vi "Settings Dialog.vi"(8 "error in (no error)":errorcluster, 11 "Settings in":T1 {"Voltage Limit" scale=0.0..155.0 scale format="%.3g"; "Hardware Configuration"."Baud Rate" items=["<0>"=0, "4800"=4800, "9600"=9600, "19200"=19200, "38400"=38400, "57600"=57600, "115200"=115200]}) -> (0 "error out":errorcluster, 1 "Cancelled?":bool, 2 "UI Refresh Needed?":bool, 3 "Settings out":T1 {"Voltage Limit" scale=0.0..155.0 scale format="%.3g"; "Hardware Configuration"."Baud Rate" items=["<0>"=0, "4800"=4800, "9600"=9600, "19200"=19200, "38400"=38400, "57600"=57600, "115200"=115200]})   [LabVIEW 2022 SP3, in "Settings.lvlib"]
doc: "Dialog for selecting user specified settings."
uses:
  Settings.lvlib
  Settings.ctl
  Acquisition/Hardware Configuration.ctl
  Logging/Logging Configuration.ctl
  <vilib>/Utility/xml.llb/Write to XML File(string).vi
  Acquisition/Acquisition.lvlib
  Logging/Logging.lvlib
panel:
  in  "Reset on Connect":bool
  in  "VISA resource name":refnum<visa-resource-name>
  in  "Baud Rate":u32(ring) items=["<0>"=0, "4800"=4800, "9600"=9600, "19200"=19200, "38400"=38400, "57600"=57600, "115200"=115200]
  in  "Cancel":bool
  in  "OK Button":bool
  # "Non visible portion of dialog (needed for connector pane)."
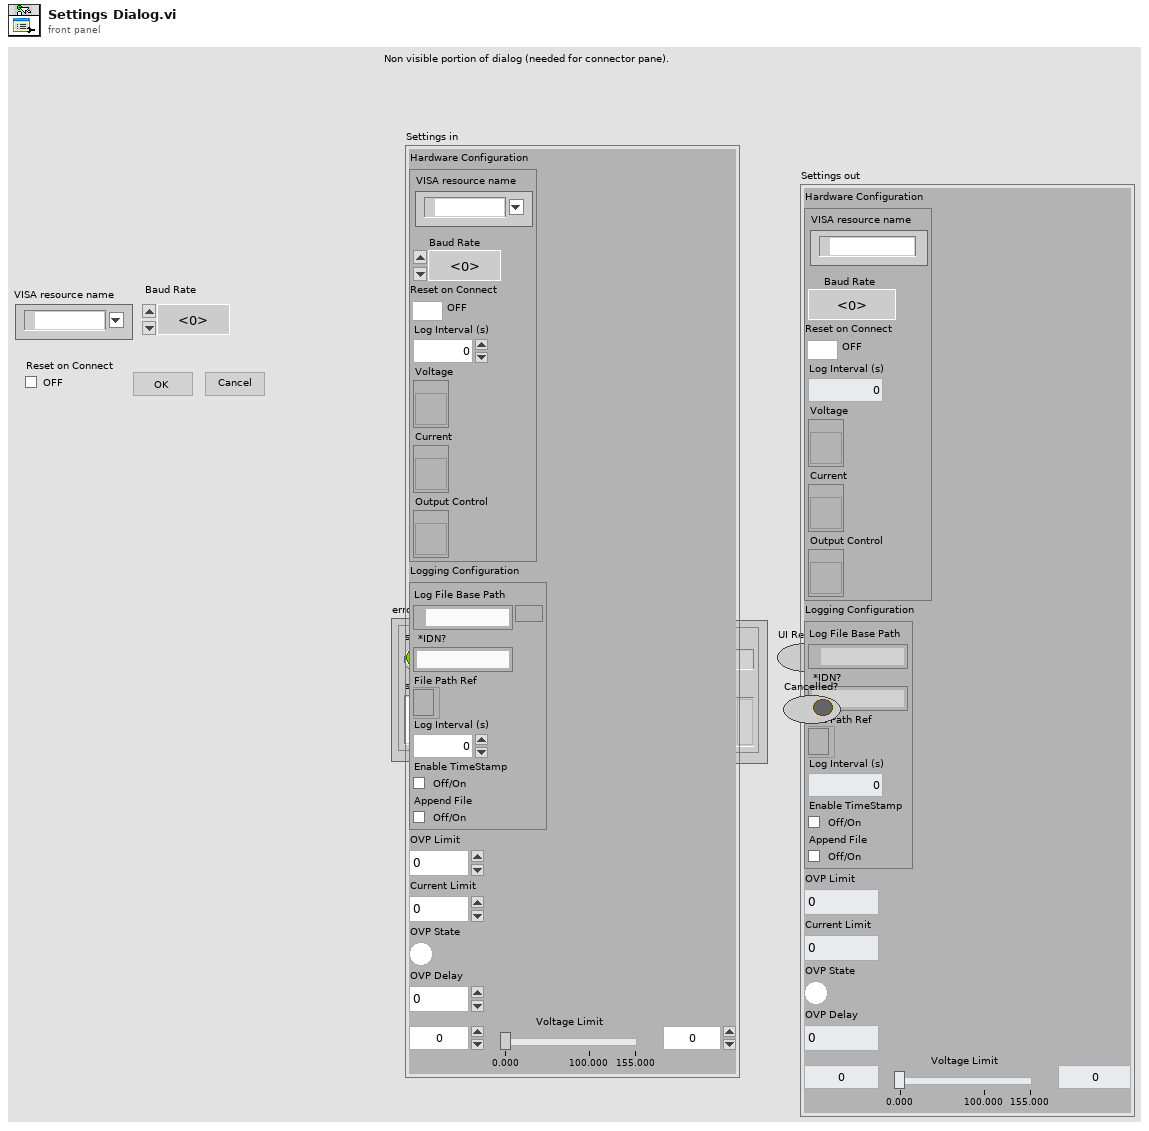
[diagram p1: front panel]
types:
  T1 = typedef "Settings.lvlib/Settings.ctl" = cluster{"Hardware Configuration":T2, "Logging Configuration":T3, "OVP Limit":dbl, "Current Limit":dbl, "OVP State":bool, "OVP Delay":dbl, "Voltage Limit":cluster{"Numeric":dbl, "Numeric":dbl}}
  T2 = typedef "Acquisition.lvlib/Hardware Configuration.ctl" = cluster{"VISA resource name":refnum<visa-resource-name>, "Baud Rate":u32, "Reset on Connect":bool, "Log Interval (s)":dbl, "Voltage":refnum<vi>, "Current":refnum<vi>, "Output Control":refnum<vi>}
  T3 = typedef "Logging.lvlib/Logging Configuration.ctl" = cluster{"Log File Base Path":path, "*IDN?":string, "File Path Ref":refnum<file>, "Log Interval (s)":dbl, "Enable TimeStamp":bool, "Append File":bool}
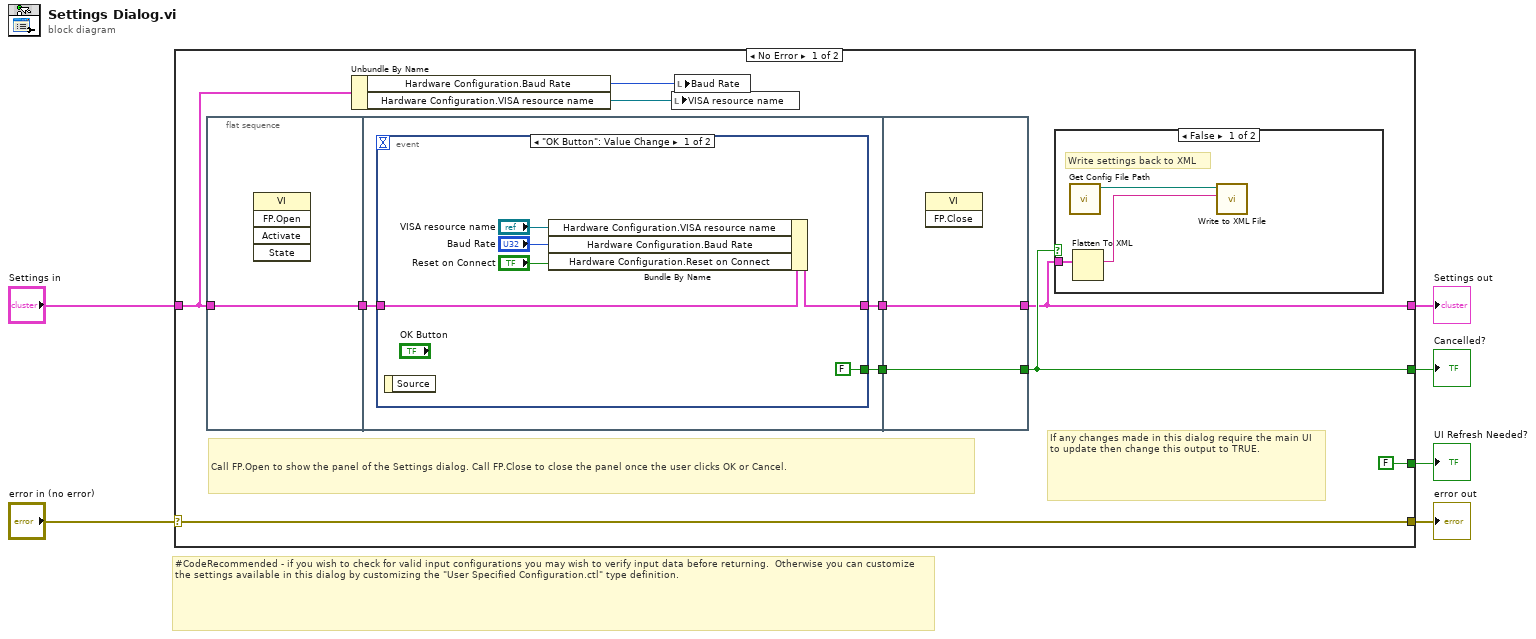
[diagram p0: block diagram]
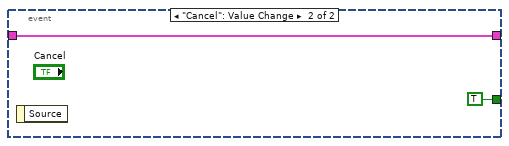
[diagram p2: hidden frame]
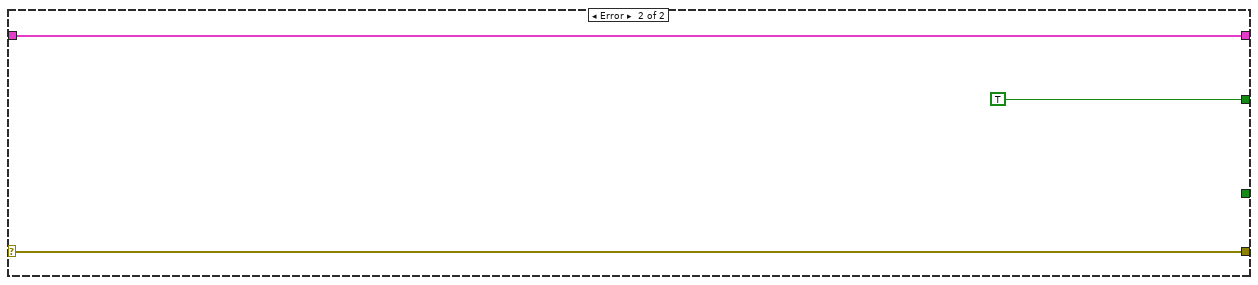
[diagram p4: hidden frame]
diagram:
  # "#CodeRecommended - if you wish to check for valid input configurations you may wish to verify input data before returning.  Otherwise you can customize the settings available in this dialog by customizing the \"User Specified Configuration.ctl\" type definition."
  n1 = case shown="No Error" "error in (no error)" {
    selector: "error in (no error)" -> [w16 w36]
    tunnel: [w16 w36] -> w5
    tunnel: "Settings in" -> [w12 w35]
    tunnel: [w13 w35] -> w3
    tunnel: [FALSE ("UI Refresh Needed?") _] -> w2
    tunnel: [w14 TRUE ("UI Refresh Needed?")] -> w1
    frame No Error {
      # "Call FP.Open to show the panel of the Settings dialog. Call FP.Close to close the panel once the user clicks OK or Cancel."
      # "If any changes made in this dialog require the main UI to update then change this output to TRUE."
      n2 = flat-sequence {
        tunnel: w12 -> [w17]
        tunnel: [w17] -> w11
        tunnel: w11 -> [w18]
        tunnel: [w20] -> w10
        tunnel: [w19] -> w9
        tunnel: [w29] -> w13
        tunnel: [w30] -> w14
        tunnel: w10 -> [w30]
        tunnel: w9 -> [w29]
        frame #0 {
          n3 = invoke class="VI" method="FP.Open"() -> ()  [unwired: 5 in, 5 out]
        }
        frame #1 {
          n4 = event shown="[0] \"OK Button\": Value Change" {
            selector: _ -> [_ _]
            dyn-events: _ -> [_ _]
            timeout: _ -> [_ _]
            tunnel: [w24 w28] -> w19
            tunnel: w18 -> [w25 w28]
            tunnel: [FALSE ("UI Refresh Needed?") TRUE ("UI Refresh Needed?")] -> w20
            event "OK Button": Value Change {
              n5 = event-data() -> ()  [unwired: 1 in, 1 out]
              n6 = Bundle By Name(cluster=w25, "Hardware Configuration.VISA resource name"="VISA resource name", "Hardware Configuration.Baud Rate"="Baud Rate", "Hardware Configuration.Reset on Connect"="Reset on Connect") -> (w24:T1)
            }
            event "Cancel": Value Change {
              n7 = event-data() -> ()  [unwired: 1 in, 1 out]
            }
          }
        }
        frame #2 {
          n8 = invoke class="VI" method="FP.Close"() -> ()  [unwired: 3 in, 3 out]
        }
      }
      n9 = Unbundle By Name(w12) -> ("Hardware Configuration.Baud Rate"=w8:u32, "Hardware Configuration.VISA resource name"=w7:refnum<visa-resource-name>)
      n10 = local write "VISA resource name"(w7) -> ()
      n11 = local write "Baud Rate"(w8) -> ()
      n12 = case shown="False" w14 {
        tunnel: w13 -> [w32 _]
        frame False {
          # "Write settings back to XML"
          n13 = call "Get Config File Path.vi"() -> ("XML File Path"=w33:path)  [unwired: 10 in, 1 out]
          n14 = Flatten To XML(6:w32) -> (2:w31:string)
          n15 = call-poly <vilib>:"Write to XML File.vi"("XML Input"=w31, "XML File Path"=w33) -> ()  [unwired: 7 in, 3 out]
        }
        frame True {
        }
      }
    }
    frame Error {
    }
  }
  "UI Refresh Needed?" <- w2
  "error out" <- w5
  "Settings out" <- w3
  "Cancelled?" <- w1
